vi "Get Profile Start Index.vi"(4 "Profile Info":T1={"Profile Cnt"=1, "Envelope"=FALSE, " Profile Data Point"=0, " X Start"=0, " X Pitch"=0}) -> (1 "Start Index[4]":u32[](array[numeric]))   [LabVIEW 2014, in "Keyence LJ-V7000.lvlib"]
uses:
  Keyence LJ-V7000.lvlib
  Public/Clusters/Profile Info.ctl
panel:
  # "Head A Max"
  # "Head B Max"
  # "Head A min"
  # "Head B Min"
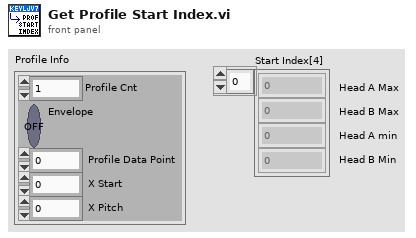
[diagram p1: front panel]
types:
  T1 = typedef "Keyence LJ-V7000.lvlib/Profile Info.ctl" = cluster{"Profile Cnt":u8, "Envelope":bool, " Profile Data Point":u16, " X Start":i32, " X Pitch":i32}
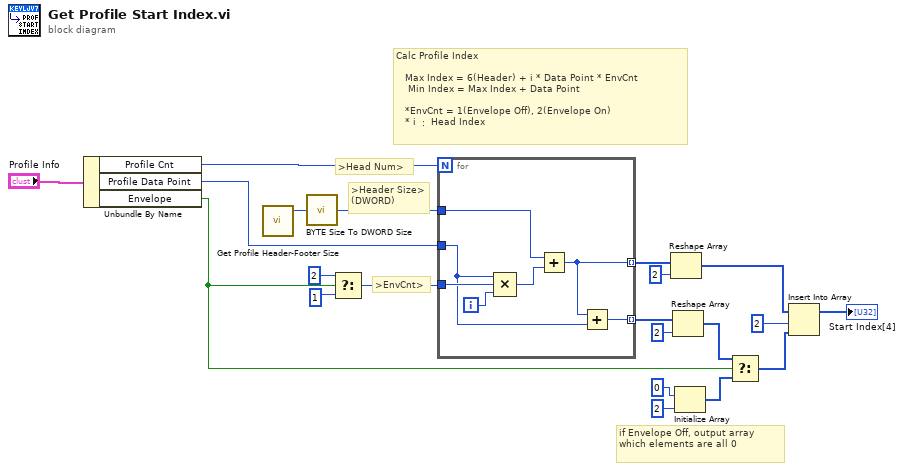
[diagram p0: block diagram]
diagram:
  # ">Head Num>"
  # ">Header Size>\n(DWORD)"
  # ">EnvCnt>"
  # "if Envelope Off, output array\nwhich elements are all 0"
  # "Calc Profile Index\n   \n   Max Index = 6(Header) + i * Data Point * EnvCnt\n　 Min Index = Max Index + Data Point\n\n　*EnvCnt = 1(Envelope Off), 2(Envelope On)\n　* i ： Head Index"
  n1 = Unbundle By Name("Profile Info") -> ("Profile Cnt"=w21:u8, "Profile Data Point"=w12:u16, "Envelope"=w7:bool)
  n2 = call "Get Profile Header-Footer Size.vi"() -> ("Header Size"=w18:u32)  [unwired: 4 in, 1 out]
  n3 = call "BYTE Size To DWORD Size.vi"("BYTE Size"=w18) -> ("DWORD Size"=w17:u32)
  n4 = Select(t=u32 2, s=w7, f=u32 1) -> (s? t:f=w13:u32)
  n5 = for {
    N: w21 -> [_]
    tunnel: w13 -> [w28]
    tunnel: w12 -> [w22]
    tunnel: w17 -> [w23]
    tunnel: [w26] -> w16 mode=indexing
    tunnel: [w25] -> w10 mode=indexing
    i -> [w27]
    n6 = Compound Arithmetic op=MULTIPLY(w22, w28, w27) -> (w24:u32)
    n7 = Add(x=w23, y=w24) -> (x+y=w26:u32)
    n8 = Add(x=w26, y=w22) -> (x+y=w25:u32)
  }
  n9 = Reshape Array(w16, 2 ("次元サイズ")) -> (w4:u32[])
  n10 = Reshape Array(w10, 2 ("次元サイズ")) -> (w6:u32[])
  n11 = Initialize Array(u32 0 ("次元サイズ"), 2 ("次元サイズ")) -> (w5:u32[])
  n12 = Select(t=w6, s=w7, f=w5) -> (s? t:f=w3:u32[])
  n13 = Insert Into Array(array=w4, index=2 ("指標"), new element=w3) -> (→"Start Index[4]":u32[])
